vi "Vision_Version_1.vi"(0 "Source Image":T1, 5 "Red or Hue":cluster{"Lower value":i32, "Upper value":i32}={"Lower value"=155, "Upper value"=245}, 7 "Green or saturation":cluster{"Lower value":i32, "Upper value":i32}={"Lower value"=148, "Upper value"=255}, 9 "Blue or luminance":cluster{"Lower value":i32, "Upper value":i32}={"Lower value"=9, "Upper value"=93}, 11 "Error in":errorcluster) -> (4 "Apply Convex Hull":T1(plugin-control), 6 "Pixel Area":dbl, 8 "Center of Mass X":dbl, 10 "Turn degrees":dbl, 14 "Positive or Negative?":dbl, 15 "error out":errorcluster)   [LabVIEW 2017]
uses:
  <vilib>/vision/Image Controls.llb/IMAQ Image.ctl
  <vilib>/vision/NI_Vision_Development_Module.lvlib
panel:
  out "sum":dbl
  out "After RGB":T1(plugin-control)
  out "Original Image":T1(plugin-control)
  out "Noise Removed":T1(plugin-control)
  out "Number of Regions":i32
  out "Particle Measurements (Pixels)":dbl[][](array[numeric]) format="%.2f"
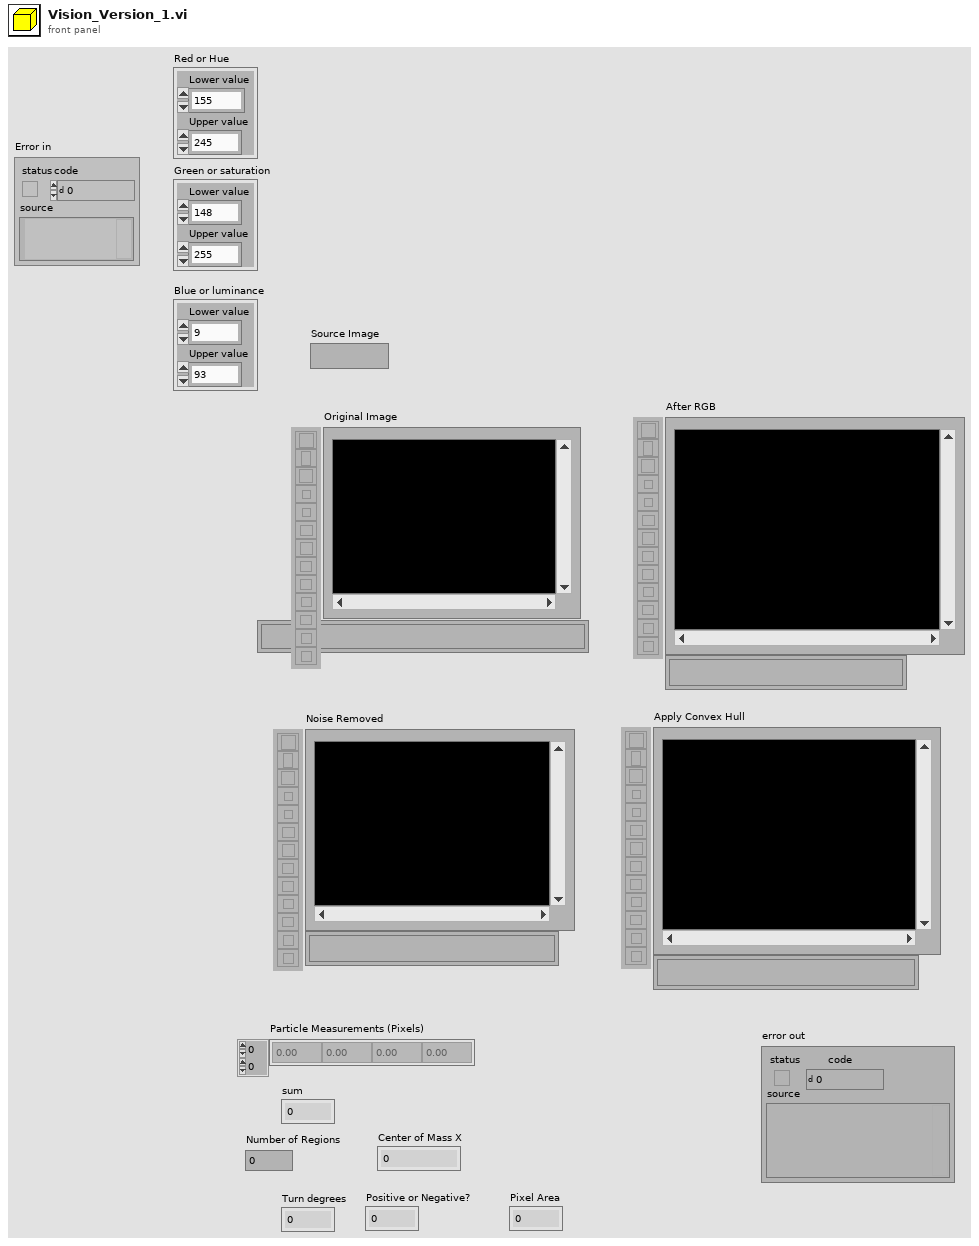
[diagram p1: front panel]
types:
  T1 = typedef "IMAQ Image.ctl" = refnum<image>
  T2 = typedef "Particle Parameters" = i32
  T3 = cluster{"Measurement Parameter":T2, dbl, dbl, bool, bool}
  T4 = cluster{"Measurement Parameter":T2, dbl, dbl, bool, bool}[]
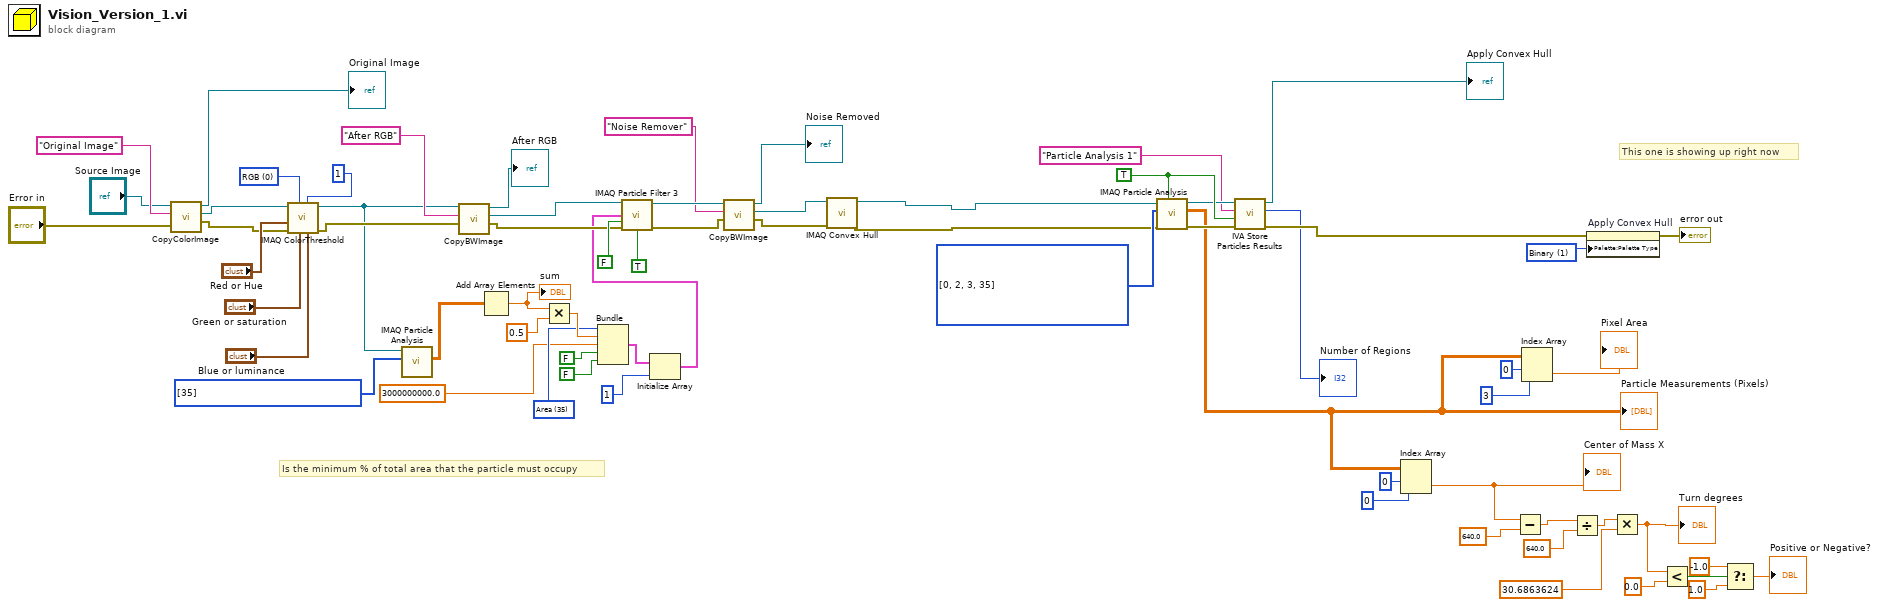
[diagram p0: block diagram]
diagram:
  w25 = T2 35 items=["Center of Mass X", "Center of Mass Y", "First Pixel X", "First Pixel Y", "Bounding Rect Left", "Bounding Rect Top", "Bounding Rect Right", "Bounding Rect Bottom", "Max Feret Diameter Start X", "Max Feret Diameter Start Y", "Max Feret Diameter End X", "Max Feret Diameter End Y", "Max Horiz. Segment Length Left", "Max Horiz. Segment Length Right", "Max Horiz. Segment Length Row", "-", "Bounding Rect Width", "Bounding Rect Height", "Bounding Rect Diagonal", "Perimeter", "Convex Hull Perimeter", "Holes' Perimeter", "Max Feret Diameter", "Equivalent Ellipse Major Axis", "Equivalent Ellipse Minor Axis", "Equivalent Ellipse Minor Axis (Feret)", "Equivalent Rect Long Side", "Equivalent Rect Short Side", "Equivalent Rect Diagonal", "Equivalent Rect Short Side (Feret)", "Average Horiz. Segment Length", "Average Vert. Segment Length", "Hydraulic Radius", "Waddel Disk Diameter", "-", "Area", "Holes' Area", "Particle & Holes' Area", "Convex Hull Area", "Image Area", "-", "Number of Holes", "Number of Horiz. Segments", "Number of Vert. Segments", "-", "Orientation", "Max Feret Diameter Orientation", "-", "% Area/Image Area", "% Area/(Particle & Holes' Area)", "Ratio of Equivalent Ellipse Axes", "Ratio of Equivalent Rect Sides", "-", "Elongation Factor", "Compactness Factor", "Heywood Circularity Factor", "Type Factor", "-", "Sum X", "Sum Y", "Sum XX", "Sum XY", "Sum YY", "Sum XXX", "Sum XXY", "Sum XYY", "Sum YYY", "-", "Moment of Inertia XX", "Moment of Inertia XY", "Moment of Inertia YY", "Moment of Inertia XXX", "Moment of Inertia XXY", "Moment of Inertia XYY", "Moment of Inertia YYY", "Norm. Moment of Inertia XX", "Norm. Moment of Inertia XY", "Norm. Moment of Inertia YY", "Norm. Moment of Inertia XXX", "Norm. Moment of Inertia XXY", "Norm. Moment of Inertia XYY", "Norm. Moment of Inertia YYY", "Hu Moment 1", "Hu Moment 2", "Hu Moment 3", "Hu Moment 4", "Hu Moment 5", "Hu Moment 6", "Hu Moment 7"] ("Measurement Parameter")
  w32 = i32[] [35] items=["Center of Mass X", "Center of Mass Y", "First Pixel X", "First Pixel Y", "Bounding Rect Left", "Bounding Rect Top", "Bounding Rect Right", "Bounding Rect Bottom", "Max Feret Diameter Start X", "Max Feret Diameter Start Y", "Max Feret Diameter End X", "Max Feret Diameter End Y", "Max Horiz. Segment Length Left", "Max Horiz. Segment Length Right", "Max Horiz. Segment Length Row", "-", "Bounding Rect Width", "Bounding Rect Height", "Bounding Rect Diagonal", "Perimeter", "Convex Hull Perimeter", "Holes' Perimeter", "Max Feret Diameter", "Equivalent Ellipse Major Axis", "Equivalent Ellipse Minor Axis", "Equivalent Ellipse Minor Axis (Feret)", "Equivalent Rect Long Side", "Equivalent Rect Short Side", "Equivalent Rect Diagonal", "Equivalent Rect Short Side (Feret)", "Average Horiz. Segment Length", "Average Vert. Segment Length", "Hydraulic Radius", "Waddel Disk Diameter", "-", "Area", "Holes' Area", "Particle & Holes' Area", "Convex Hull Area", "Image Area", "-", "Number of Holes", "Number of Horiz. Segments", "Number of Vert. Segments", "-", "Orientation", "Max Feret Diameter Orientation", "-", "% Area/Image Area", "% Area/(Particle & Holes' Area)", "Ratio of Equivalent Ellipse Axes", "Ratio of Equivalent Rect Sides", "-", "Elongation Factor", "Compactness Factor", "Heywood Circularity Factor", "Type Factor", "-", "Sum X", "Sum Y", "Sum XX", "Sum XY", "Sum YY", "Sum XXX", "Sum XXY", "Sum XYY", "Sum YYY", "-", "Moment of Inertia XX", "Moment of Inertia XY", "Moment of Inertia YY", "Moment of Inertia XXX", "Moment of Inertia XXY", "Moment of Inertia XYY", "Moment of Inertia YYY", "Norm. Moment of Inertia XX", "Norm. Moment of Inertia XY", "Norm. Moment of Inertia YY", "Norm. Moment of Inertia XXX", "Norm. Moment of Inertia XXY", "Norm. Moment of Inertia XYY", "Norm. Moment of Inertia YYY", "Hu Moment 1", "Hu Moment 2", "Hu Moment 3", "Hu Moment 4", "Hu Moment 5", "Hu Moment 6", "Hu Moment 7"] ("Pixel Measurements")
  w34 = u16 0 items=["RGB", "HSL", "HSV", "HSI"] ("Color Mode")
  w59 = u32 1 items=["Grayscale", "Binary", "Gradient", "Rainbow", "Temperature", "User Defined", "Binary 16 Bit", "Gradient 16 Bit", "Rainbow 16 Bit", "Temperature 16 Bit", "User Defined 16 Bit"] ("Palette Type")
  w66 = i32[] [0, 2, 3, 35] items=["Center of Mass X", "Center of Mass Y", "First Pixel X", "First Pixel Y", "Bounding Rect Left", "Bounding Rect Top", "Bounding Rect Right", "Bounding Rect Bottom", "Max Feret Diameter Start X", "Max Feret Diameter Start Y", "Max Feret Diameter End X", "Max Feret Diameter End Y", "Max Horiz. Segment Length Left", "Max Horiz. Segment Length Right", "Max Horiz. Segment Length Row", "-", "Bounding Rect Width", "Bounding Rect Height", "Bounding Rect Diagonal", "Perimeter", "Convex Hull Perimeter", "Holes' Perimeter", "Max Feret Diameter", "Equivalent Ellipse Major Axis", "Equivalent Ellipse Minor Axis", "Equivalent Ellipse Minor Axis (Feret)", "Equivalent Rect Long Side", "Equivalent Rect Short Side", "Equivalent Rect Diagonal", "Equivalent Rect Short Side (Feret)", "Average Horiz. Segment Length", "Average Vert. Segment Length", "Hydraulic Radius", "Waddel Disk Diameter", "-", "Area", "Holes' Area", "Particle & Holes' Area", "Convex Hull Area", "Image Area", "-", "Number of Holes", "Number of Horiz. Segments", "Number of Vert. Segments", "-", "Orientation", "Max Feret Diameter Orientation", "-", "% Area/Image Area", "% Area/(Particle & Holes' Area)", "Ratio of Equivalent Ellipse Axes", "Ratio of Equivalent Rect Sides", "-", "Elongation Factor", "Compactness Factor", "Heywood Circularity Factor", "Type Factor", "-", "Sum X", "Sum Y", "Sum XX", "Sum XY", "Sum YY", "Sum XXX", "Sum XXY", "Sum XYY", "Sum YYY", "-", "Moment of Inertia XX", "Moment of Inertia XY", "Moment of Inertia YY", "Moment of Inertia XXX", "Moment of Inertia XXY", "Moment of Inertia XYY", "Moment of Inertia YYY", "Norm. Moment of Inertia XX", "Norm. Moment of Inertia XY", "Norm. Moment of Inertia YY", "Norm. Moment of Inertia XXX", "Norm. Moment of Inertia XXY", "Norm. Moment of Inertia XYY", "Norm. Moment of Inertia YYY", "Hu Moment 1", "Hu Moment 2", "Hu Moment 3", "Hu Moment 4", "Hu Moment 5", "Hu Moment 6", "Hu Moment 7"] ("Pixel Measurements")
  w65 = TRUE ("Connectivity 4/8 (8)")
  # "Is the minimum % of total area that the particle must occupy"
  # "This one is showing up right now"
  n1 = call "CopyColorImage.vi"("Error in 1"="Error in", "Image Name"="Original Image", "Image"="Source Image") -> ("error out 2"=w36:errorcluster, "Out 2"=w49:T1, "Out"=→"Original Image":T1)  [unwired: 5 in, 1 out]
  n2 = call "IMAQ ColorThreshold"("Blue or Luma or Val or Inten Range"="Blue or luminance", "Replace Value"=1, "Green or Sat Range"="Green or saturation", "Color Mode"=w34, "error in (no error)"=w36, "Red or Hue Range"="Red or Hue", "Image Src"=w49) -> ("error out"=w44:errorcluster, "Image Dst Out"=w33:T1)  [unwired: 1 in, 2 out]
  n3 = call "IMAQ Particle Analysis"("Pixel Measurements"=w32, "Image"=w33) -> ("Particle Measurements (Pixels)"=w31:dbl[][])  [unwired: 3 in, 6 out]
  n4 = call "CopyBWImage.vi"("Error in 1"=w44, "Image Name"="After RGB", "Image"=w33) -> ("error out 2"=w47:errorcluster, "Out 2"=w48:T1, "Out"=→"After RGB":T1)  [unwired: 5 in, 1 out]
  n5 = Add Array Elements(numeric array=w31) -> (sum=w30:dbl)
  "sum" <- w30
  n6 = Multiply(x=w30, y=0.5) -> (x*y=w28:dbl)
  n7 = Bundle("Measurement Parameter"=w25, w28, 3000000000.0, FALSE, FALSE) -> (w27:T3)  [unwired: 1 in]
  n8 = Initialize Array(w27, 1 ("dimension size")) -> (w21:T4)
  n9 = call "IMAQ Particle Filter 3"("Image Src"=w48, "Selection Values"=w21, "Keep/Remove Particles (F)"=FALSE, "error in (no error)"=w47, "Fill Holes? (F)"=TRUE) -> ("Image Dst Out"=w41:T1, "error out"=w40:errorcluster)  [unwired: 8 in, 1 out]
  n10 = call "CopyBWImage.vi"("Error in 1"=w40, "Image Name"="Noise Remover", "Image"=w41) -> ("error out 2"=w42:errorcluster, "Out 2"=w43:T1, "Out"=→"Noise Removed":T1)  [unwired: 5 in, 1 out]
  n11 = call "IMAQ Convex Hull"("error in (no error)"=w42, "Image Src"=w43) -> ("error out"=w51:errorcluster, "Image Dst Out"=w52:T1)  [unwired: 8 in]
  n12 = call "IMAQ Particle Analysis"("Connectivity 4/8 (8)"=w65, "error in (no error)"=w51, "Pixel Measurements"=w66, "Image"=w52) -> ("error out"=w62:errorcluster, "Particle Measurements (Pixels)"=w6:dbl[][], "Image Out (duplicate)"=w64:T1)  [unwired: 1 in, 4 out]
  "Particle Measurements (Pixels)" <- w6
  n13 = call <vilib>:"IVA Store Particles Results.vi"("error in (no error)"=w62, "Connectivity 4/8 (8)"=w65, "Step Name"="Particle Analysis 1", "Image in"=w64) -> ("error out"=w61:errorcluster, "Number of Particles"=→"Number of Regions":i32, "Image dup"=→"Apply Convex Hull":T1)  [unwired: 5 out]
  n14 = Index Array(array=w6, index (row)=0, index (col)=0 ("disabled index (col)")) -> (element=w18:dbl)
  "Center of Mass X" <- w18
  n15 = Subtract(x=w18, y=640.0) -> (x-y=w16:dbl)
  n16 = Index Array(array=w6, index (row)=0, index (col)=3 ("disabled index (col)")) -> (element=→"Pixel Area":dbl)
  n17 = Divide(x=w16, y=640.0) -> (x/y=w14:dbl)
  n18 = property on="Apply Convex Hull" class="ImageControl"(error in=w61, "Palette:Palette Type"=w59) -> (error out=→"error out":errorcluster)  [unwired: 1 in, 1 out]
  n19 = Multiply(x=w14, y=30.6863624) -> (x*y=w11:dbl)
  "Turn degrees" <- w11
  n20 = Less?(x=w11, y=0.0) -> (x < y?=w12:bool)
  n21 = Select(t=-1.0, s=w12, f=1.0) -> (s? t:f=→"Positive or Negative?":dbl)
